vi "redraw_graphs.vi"(8 "error in (no error)":errorcluster, 11 "dict of HIS IN":variant) -> (0 "error out":errorcluster, 3 "dict of HIS OUT":variant)   [LabVIEW 2015]
uses:
  cluster_template.ctl
  Classes/DATA/HIS/HIS.lvclass
  Classes/DATA/HIS/HIS.lvclass/HIS.ctl
  Classes/DATA/DATA.lvclass/DATA.ctl
  Classes/DATA/DATA.lvclass
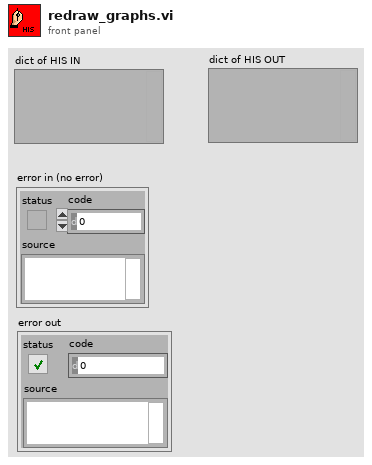
[diagram p1: front panel]
types:
  T1 = typedef "cluster_template.ctl" = cluster{"HIS.lvclass":refnum<class "HIS.lvclass">, "selector":refnum<vi>, "HIS graph":refnum<vi>, "DAT graph":refnum<vi>, "path":refnum<vi>, "path MAIN":refnum<vi>, "#":refnum<vi>, "unsel Graph":refnum<vi>, "DATgraph":refnum<vi>}
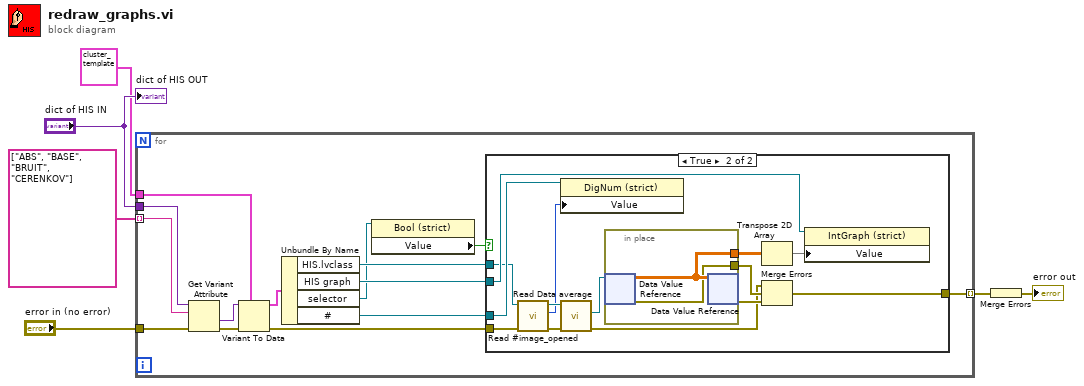
[diagram p0: block diagram]
diagram:
  n1 = for {
    tunnel: string[] ["ABS", "BASE", "BRUIT", "CERENKOV"] ("Array") -> [w16] mode=indexing
    tunnel: "dict of HIS IN" -> [w17]
    tunnel: T1 {"HIS.lvclass"=refnum, "selector"=refnum, "HIS graph"=refnum, "DAT graph"=refnum, "path"=refnum, "path MAIN"=refnum, "#"=refnum, "unsel Graph"=refnum, "DATgraph"=refnum} ("output cluster") -> [w15]
    tunnel: "error in (no error)" -> [w9]
    tunnel: [w8] -> w2 mode=indexing
    n2 = Get Variant Attribute(Variant=w17, name=w16, error in=w9) -> (value=w18:variant, error out=w20:errorcluster)  [unwired: 1 in, 2 out]
    n3 = Variant To Data(error in=w20, type=w15, Variant=w18) -> (data=w14:T1, error out=w19:errorcluster)
    n4 = Unbundle By Name(w14) -> ("HIS.lvclass"=w13:refnum<class "HIS.lvclass">, "HIS graph"=w12:refnum<vi>, "selector"=w11:refnum<vi>, "#"=w7:refnum<vi>)
    n5 = property class="Bool (strict)"(reference=w11) -> ("Value"=w10:bool)  [unwired: 1 in, 2 out]
    n6 = case shown="True" w10 {
      tunnel: w19 -> [w21 w24]
      tunnel: w13 -> [_ w26]
      tunnel: w12 -> [_ w34]
      tunnel: [w21 w30] -> w8
      tunnel: w7 -> [_ w27]
      frame False {
      }
      frame True {
        n7 = call "Read #image_opened.vi"("error in (no error)"=w24, "HIS in"=w26) -> ("error out"=w23:errorcluster, "#image_opened"=w22:i32, "HIS out"=w25:refnum<class "HIS.lvclass">)  [unwired: 7 in]
        n8 = property on="Property Node" class="DigNum (strict)"(reference=w27, "Value"=w22) -> ()  [unwired: 1 in, 2 out]
        n9 = call "Read Data average.vi"("error in (no error)"=w23, "DATA in"=w25) -> ("error out"=w31:errorcluster, "Data average"=w35:refnum<data-value>)  [unwired: 7 in, 1 out]
        n10 = in-place {
          in-place-border: [w37] -> w29
          in-place-border: [w36] -> w32
          n11 = in-place-dvr #1(w35) -> (w37:dbl[][], w36:errorcluster)
          n12 = in-place-dvr #1(w37) -> (w33:errorcluster)  [unwired: 1 out]
        }
        n13 = Transpose 2D Array(2D array=w29) -> (transposed array=w28:dbl[][])
        n14 = Merge Errors(w31, w32, w33) -> (w30:errorcluster)
        n15 = property on="Property Node" class="IntGraph (strict)"(reference=w34, "Value"=w28) -> ()  [unwired: 1 in, 2 out]
      }
    }
  }
  n16 = Merge Errors(w2) -> (→"error out":errorcluster)
  "dict of HIS OUT" <- "dict of HIS IN"
